vi "FTW-Endpoint-Multipart-Tell.vi"(0 "FTW Endpoint":refnum<class "FTW-Endpoint.lvclass">, 5 "Multipart Message":string[](array[string]), 7 "Timeout":i32 format="%dmsec", 11 "error in":errorcluster) -> (4 "FTW Endpoint out":refnum<class "FTW-Endpoint.lvclass">, 6 "Timed out?":bool, 15 "error out":errorcluster)   [LabVIEW 2012, in "FTW-Actor.lvlib" / "FTW-Endpoint.lvclass"]
uses:
  FTW-Endpoint.lvclass
  FTW-Endpoint.lvclass/FTW-Endpoint.ctl
panel:
  # "Inputs"
  # "Outputs"
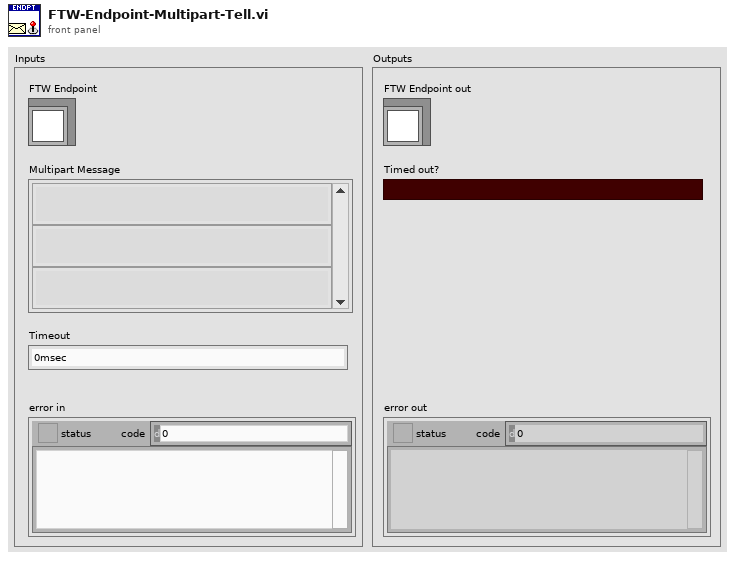
[diagram p1: front panel]
types:
  T1 = typedef "FTW-Actor.lvlib/FTW-Actor-Address.ctl" = string
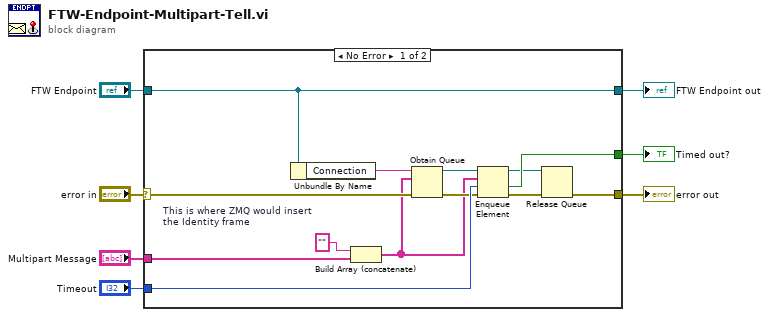
[diagram p0: block diagram]
diagram:
  n1 = case shown="No Error" "error in" {
    selector: "error in" -> [w17 w22]
    tunnel: [w11 w22] -> w7
    tunnel: [w18 w21] -> w5
    tunnel: "FTW Endpoint" -> [w18 w21]
    tunnel: "Multipart Message" -> [w10 _]
    tunnel: [w20 _] -> w2
    tunnel: "Timeout" -> [w19 _]
    frame No Error {
      w8 = ""  # This is where ZMQ would insert the Identity frame
      n2 = Unbundle By Name(w18) -> ("Connection"=w14:T1)
      n3 = Build Array (concatenate)(w8, w10) -> (w9:string[])
      n4 = Obtain Queue(name (unnamed)=w14, element data type=w9, error in (no error)=w17) -> (queue out=w15:refnum<queue>, error out=w16:errorcluster)  [unwired: 2 in, 1 out]
      n5 = Enqueue Element(queue=w15, element=w9, timeout in ms (-1)=w19, error in (no error)=w16) -> (queue out=w13:refnum<queue>, timed out?=w20:bool, error out=w12:errorcluster)
      n6 = Release Queue(queue=w13, error in (no error)=w12) -> (error out=w11:errorcluster)  [unwired: 1 in, 2 out]
    }
    frame Error {
    }
  }
  "error out" <- w7
  "FTW Endpoint out" <- w5
  "Timed out?" <- w2
